vi "AxisControl.vi"() -> ()   [LabVIEW 2020]
uses:
  <vilib>/Utility/miscctls.llb/LVTextColorsTypeDef.ctl
  AxisConfiguration_typedef.ctl
  <vilib>/Modbus/subvis/Modbus API/Modbus API.lvclass/Modbus API.ctl
  <vilib>/Modbus/subvis/Transmission Data Unit (ADU)/Transmission Data Unit/Transmission Data Unit.lvclass/Transmission Data Unit.ctl
  <vilib>/Modbus/master/Data Access/Unit ID/Set Unit ID Property.vi
  <vilib>/Modbus/subvis/Transmission Data Unit (ADU)/Transmission Data Unit/Data Access/Unit ID/Write Unit ID.vi
  <vilib>/Modbus/subvis/Modbus API/Read Transmission Data Unit.vi
  <vilib>/Modbus/subvis/Modbus API/Write Transmission Data Unit.vi
  <vilib>/Modbus/master/Modbus Master.lvclass
  C:/Program Files (x86)/National Instruments/LabVIEW 2020/vi.lib/Modbus/subvis/Modbus API/Modbus API.lvclass
  ConnectionData.vi
  AxisReadValues_Write.vi
  AxisConfiguration.vi
  AxisConfiguration_Write.vi
  AxisWriteValues.vi
  ConnectionData_Write.vi
  AxisReadValues.vi
  <vilib>/Utility/config.llb/Read Key (String).vi
  AxisWriteValues_Write.vi
  <vilib>/Utility/config.llb/Read Key (U32).vi
  <vilib>/Modbus/master/Create Master Instance (Serial).vi
  <vilib>/Modbus/master/Create Master Instance (TCP).vi
  <vilib>/Utility/config.llb/Write Key (String).vi
  <vilib>/Modbus/subvis/Transmission Data Unit (ADU)/Transmission Data Unit/Transmission Data Unit.lvclass
  SMCD14_lib.lvlib
  <vilib>/Utility/config.llb/NI_LVConfig.lvlib
panel:
  out "TimeOut value":u32
  in  "ConnectBtn2":bool
  out "ConnectionStatusIndicator":string="Not connected" caption="Connection status:"
  in  "StopAppBtn":bool caption="Close"
  in  "MainTabs":enum32{"Axis", "Connection", "Config."}(tab)
  out "AxisVelIndicator":sgl caption="Velocity [mm/s]" format="%.4g"
  out "MotorIndicator":bool caption="Motor ON"
  in  "ClearBtn":bool
  in  "StopBtn":bool caption="Stop"
  in  "RunBtn":bool caption="Run"
  in  "VelocityControl":dbl=1.0 caption="Target velocity" min=-50.0 max=50.0 step=1.0
  in  "TargetControl":dbl caption="Target position"
  in  "MoveModeControl":u16(ring)=4 caption="Movement mode" items=["Absolute"=1, "Relative"=2, "Velocity"=3, "Homing"=4, "none"=0]
  out "ErrorCodeIndicator":string="No error" caption="Error description"
  out "AxisPosIndicator":sgl caption="Position [mm]" format="%.4f"
  in  "MotorONBtn":bool
  in  "MotorOFFBtn":bool
  out "IsHomedIndicator":bool caption="Homed"
  out "IsRunningIndicator":bool caption="Running"
  out "FLSIndicator":bool caption="FLS (limit+)"
  out "BLSIndicator":bool caption="BLS (limit-)"
  out "InPosIndicator":bool caption="In position"
  out "EnabledIndicator":bool caption="Enabled"
  out "ErrorIndicator":bool caption="Error"
  out "RefIndicator":bool caption="Ref. signal"
  in  "ReadOnlyMode":bool
  in  "CheckProg":bool
  in  "BaudrateCtrl":u16=38400 caption="Baud rate"
  in  "IPCtrl":string caption="IP address"
  in  "ConnectBtn":bool
  in  "COMportCtrl":refnum<visa-resource-name> caption="COM port"
  in  "ProtocolCtrl":u16(ring) caption="Protocol" items=["Serial", "TCP/IP"]
  in  "DeviceIDCtrl":u16=1 caption="Device ID"
  in  "IsSubPanel":bool
  in  "default config file":string="defaults.ini"
  in  "SubPanelNo":u16=1 caption="SubPanelNo (0-5)"
  in  "Joystick control":bool
  in  "LogIn":bool
  in  "AxisName":string caption="Axis name"
  in  "WriteFileBtn":bool caption="Run"
  in  "ReadFileBtn":bool caption="Run"
  in  "WriteConfBtn":bool caption="Run"
  in  "ReadConfBtn":bool caption="Run"
  in  "UnitsControl":u16(ring) caption="Units" items=["mm", "°"]
  in  "AccDeccControl":dbl=30.0 caption="Acc./dec."
  in  "HomingVelControl":dbl=1.0 caption="Homing velocity"
  in  "OffsetControl":dbl caption="Offset"
  in  "GainControl":dbl=1.0 caption="Gain (gear)"
  in  "BacklashControl":dbl=0.1 caption="Backlash distance"
  in  "HomingTypeControl":u16(ring)=4 caption="Homing type" items=["no homing"=0, "forward limit switch"=1, "backward limit switch"=2, "forward reference"=4, "backward reference"=8]
  in  "JoyMaxSpeed":dbl caption="Joystick max speed"
  in  "JoyMinSpeed":dbl caption="Joystick min. speed"
  in  "Max Velocity":dbl caption="Max. Velocity"
  # "Advanced"
  # "Display settings"
  # "Device settings"
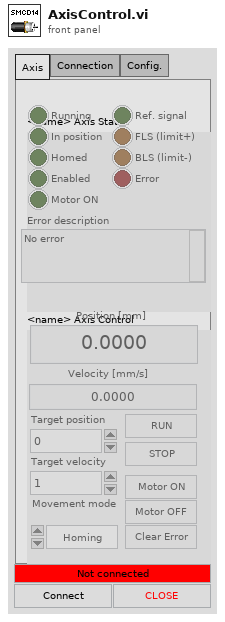
[diagram p1: front panel]
types:
  T1 = typedef "NI_LVConfig.lvlib/Config Data RefNum.ctl" = refnum<k1>
  T2 = typedef "SMCD14_lib.lvlib/AxisConfiguration_typedef.ctl" = cluster{"AxisHomeType":u16, "AxisBacklash":dbl, "AxisGain":dbl, "AxisOffset":dbl, "AxisUnit":u16, "ReqConfRead":bool, "ReqConfWrite":bool, "AxisName":string, "AxisAccDecc":dbl, "AxisHomeVel":dbl}
  T3 = cluster{"Joy_slow_speed":sgl, "Joy_slow_fast":sgl, "Name":string, "UnitsControl":u16, "MaxVel":sgl, "Joystick_control":bool}
  T4 = cluster{"DeviceIDCtrl":u16, "ProtocolCtrl":enum16{"Modbus RTU", "Modbus TCP", ""}, "COMportCtrl":refnum<visa-resource-name>, "IPCtrl":string}
  T5 = typedef "SMCD14_lib.lvlib/AxisWriteValues_typedef.ctl" = cluster{"AxisTarget":dbl, "AxisTargetVel":dbl, "AxisStartReq":bool, "AxisStopReq":bool, "AxisClearReq":bool, "AxisMovetype":bool, "AxisMotorON":bool, "MoveModeControl":u16, "AxisHomingVel":dbl, "AxisAccDecc":dbl}
  T6 = enum8{"Enabled", "Disabled", "Disabled and Grayed Out"}
  T7 = cluster{"Joy_slow_speed":dbl, "Joy_slow_fast":dbl, "Name":string, "UnitsControl":u16, "MaxVel":dbl}
  T8 = typedef "SMCD14_lib.lvlib/ConnectionData_typedef.ctl" = cluster{"DeviceIDCtrl":u16, "ProtocolCtrl":enum16{"Modbus RTU", "Modbus TCP", ""}, "COMportCtrl":refnum<visa-resource-name>, "IPCtrl":string, "serial master instance":refnum<class "Modbus Master.lvclass">, "ConnectionStatusIndicator":bool}
  T9 = typedef "SMCD14_lib.lvlib/AxisReadValues_typedef.ctl" = cluster{"AxisPosition":dbl, "AxisStatus":i16, "AxisErrorCode":i16, "AxisInPos":bool, "AxisRun":bool, "AxisHomed":bool, "AxisFLS":bool, "AxisBLS":bool, "AxisEnabled":bool, "AxisError":bool, "AxisDog":bool, "AxisVelocity":dbl, "AxisHeartbeat":i16, "SICStatus":i16, "AxisMotorON":bool}
  T10 = enum32{"invalid app kind", "Development System", "Run Time System", "Student Edition", "Embedded LabVIEW", "Evaluation", "Custom"}
  T11 = typedef "LVTextColorsTypeDef.ctl" = cluster{"Text Color":u32, "Background Color":u32}
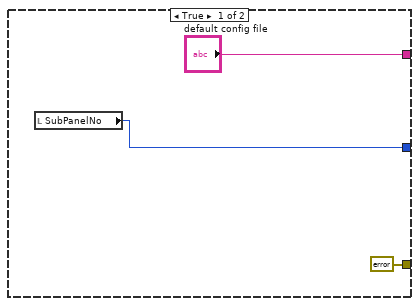
[diagram p2: hidden frame]
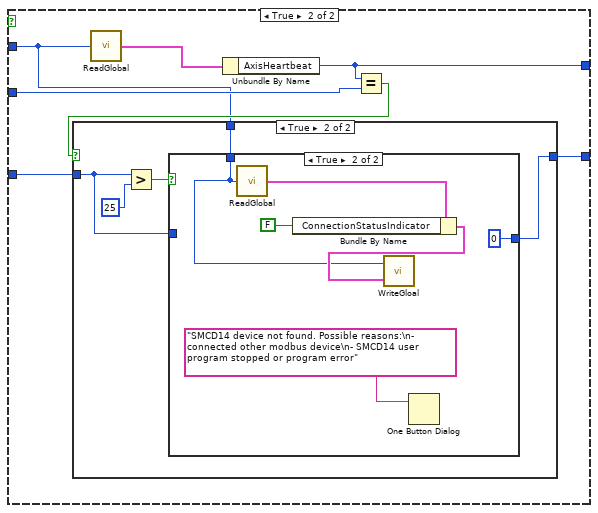
[diagram p3: hidden frame]
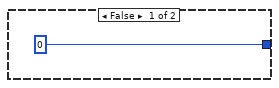
[diagram p4: hidden frame]
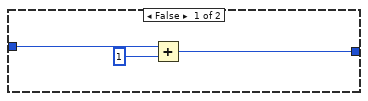
[diagram p5: hidden frame]
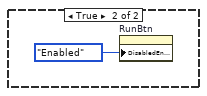
[diagram p6: hidden frame]
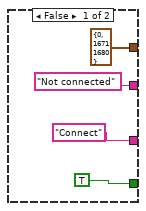
[diagram p7: hidden frame]
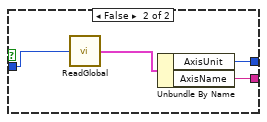
[diagram p8: hidden frame]
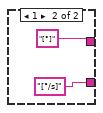
[diagram p9: hidden frame]
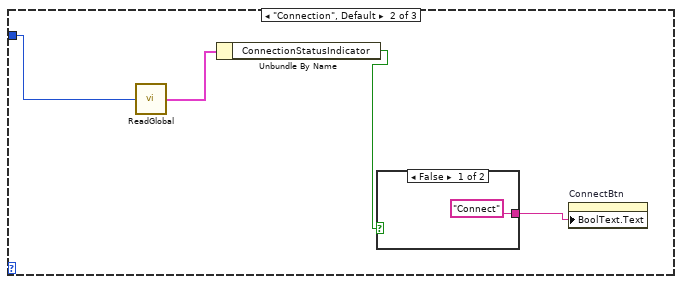
[diagram p10: hidden frame]
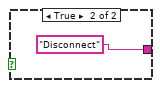
[diagram p11: hidden frame]
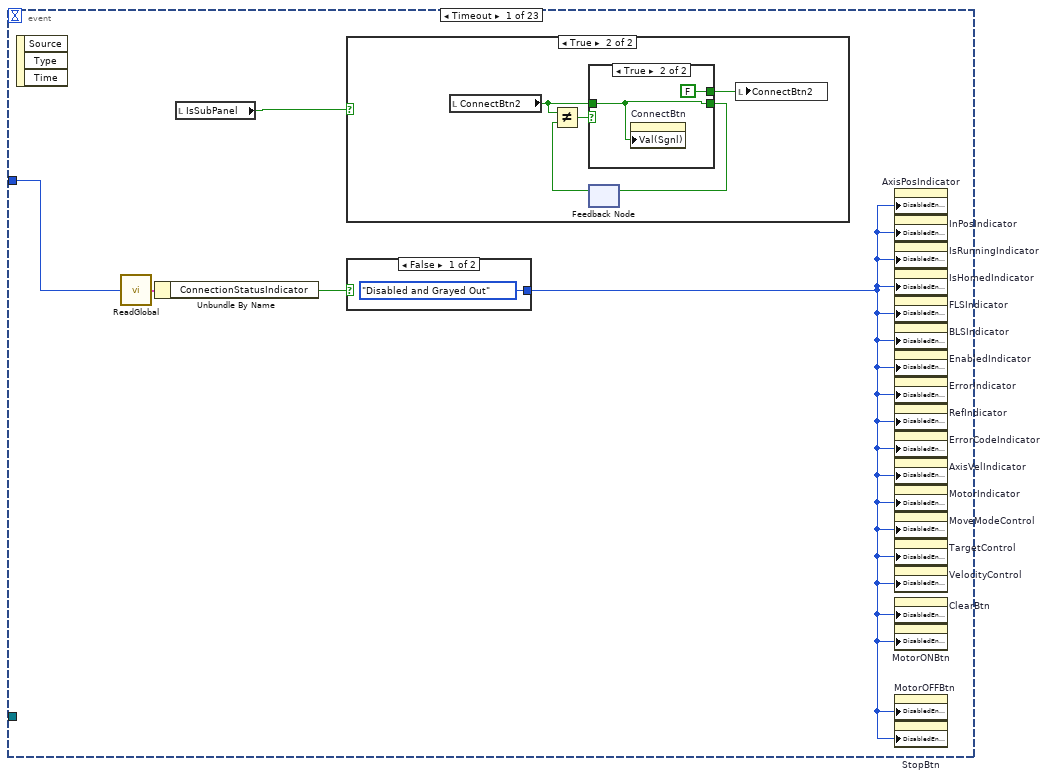
[diagram p13: hidden frame]
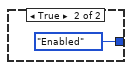
[diagram p14: hidden frame]
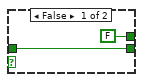
[diagram p16: hidden frame]
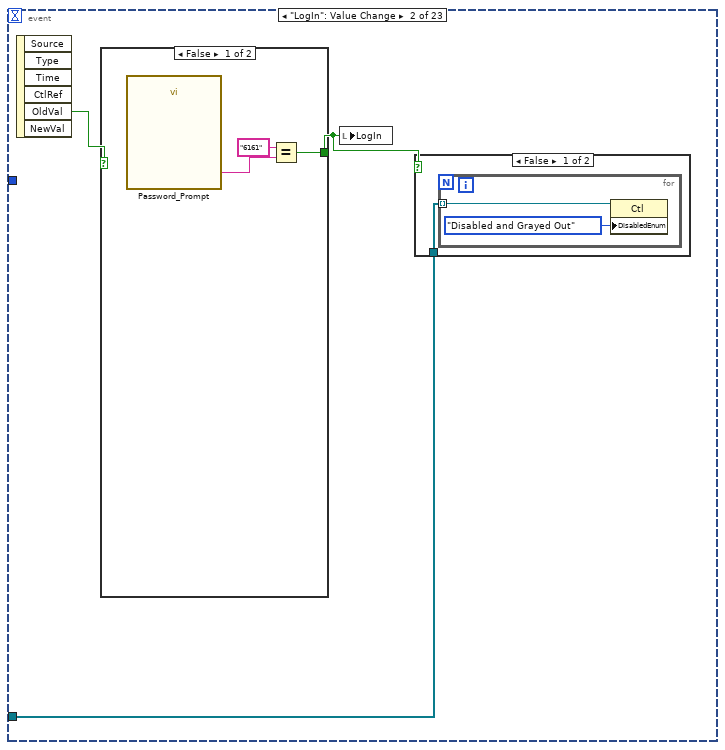
[diagram p17: hidden frame]
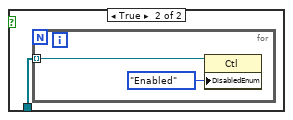
[diagram p18: hidden frame]
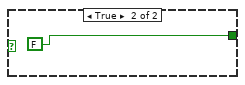
[diagram p19: hidden frame]
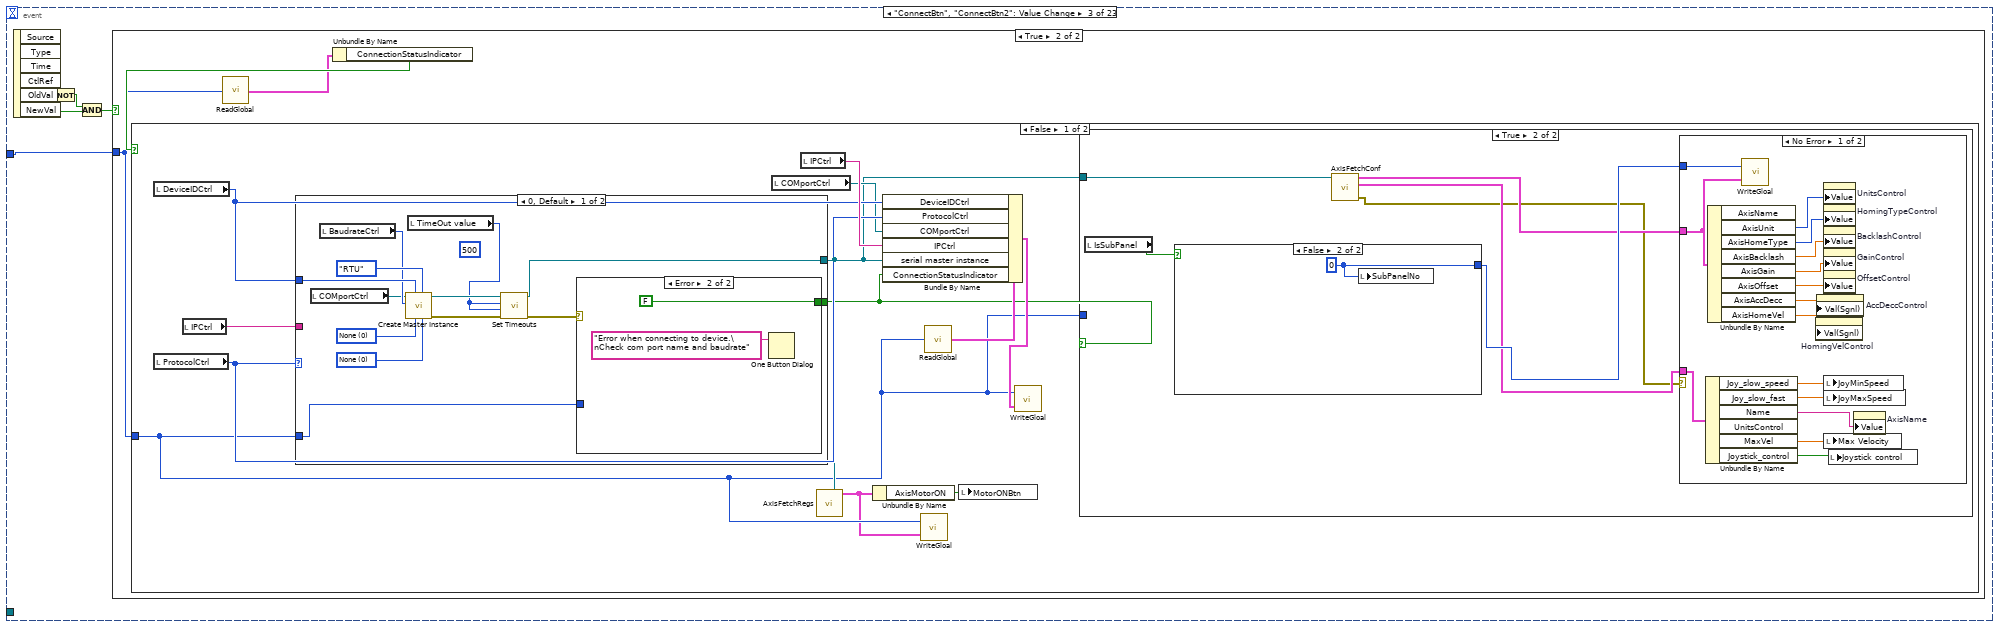
[diagram p20: hidden frame]
diagram:
  # "Wczytanie ustawień domyślnych z pliku defaults.ini w aktualnym folderze"
  # "Wspólne"
  # "Zakładka Configuration"
  # "Zakładka Axis"
  # "Zakładka Connection"
  n1 = local read "IsSubPanel"() -> (w4:bool)
  n2 = case shown="False" w4 {
    tunnel: ["default config file" w41] -> w13
    tunnel: [errorcluster {"status"=FALSE, "code"=0, "source"=""} ("error out") w38] -> w12
    tunnel: [w33 w36] -> w3
    frame True {
      n3 = local read "SubPanelNo"() -> (w33:u16)
    }
    frame False {
      w36 = 0
      n4 = call <vilib>:"Application Directory.vi"() -> ("Application Directory"=w48:path)
      n5 = local write "SubPanelNo"(w36) -> ()
      n6 = Build Path(base path=w48, name or relative path="SMCD14AxisControl.ini") -> (appended path=w46:path)
      n7 = call <vilib>:"Open Config Data.vi"("create file if necessary (T)"=TRUE, "configuration file path"=w46) -> ("error out"=w37:errorcluster, "refnum"=w45:T1)  [unwired: 7 in, 1 out]
      n8 = call-poly <vilib>:"Read Key.vi"("section"="default", "error in (no error)"=w37, "default value"="defaults.ini", "key"="ConfigFile", "refnum"=w45) -> ("error out"=w39:errorcluster, "value"=w41:string, "refnum out"=w40:T1)  [unwired: 3 in, 1 out]
      n9 = call <vilib>:"Close Config Data.vi"("error in (no error)"=w39, "refnum"=w40) -> ("error out"=w38:errorcluster)  [unwired: 8 in, 1 out]
    }
  }
  n10 = Not(x=w4) -> (.not. x?=w2:bool)
  n11 = property on="StopAppBtn" class="Bool (strict)"("Visible"=w2) -> ()  [unwired: 2 in, 2 out]
  n12 = property on="ConnectBtn2" class="Bool (strict)"("Visible"=w2) -> ()  [unwired: 2 in, 2 out]
  n13 = flat-sequence {
    tunnel: w13 -> [w76]
    tunnel: w12 -> [w75]
    tunnel: [w74] -> w11
    tunnel: [w60] -> w5
    tunnel: w3 -> [w52]
    frame #0 {
      n14 = call <vilib>:"Application Directory.vi"() -> ("Application Directory"=w79:path)
      n15 = call <vilib>:"Clear Errors.vi"("error in (no error)"=w75) -> ()  [unwired: 5 in, 2 out]
      n16 = Build Path(base path=w79, name or relative path=w76) -> (appended path=w74:path)
      n17 = call-poly "ReadGlobal.vi"("AxisNo"=w52) -> ("AxisConfigurationOUT"=w57:T2)
      n18 = call "AxisGetConfFromFile.vi"("conf file path"=w74, "AxisConfigurationIn"=w57) -> ("error out"=w60:errorcluster, "AditionalConfigOut"=w73:T3, "AxisConfigurationOut"=w56:T2, "Comunication"=w51:T4)  [unwired: 5 in, 1 out]
      n19 = call-poly "WriteGloal.vi"("AxisConfigurationIN"=w56, "AxisNo"=w52) -> ()  [unwired: 1 in]
      n20 = Unbundle By Name(w73) -> ("Joy_slow_speed"=w59:sgl, "Joy_slow_fast"=w58:sgl, "MaxVel"=w66:sgl, "Joystick_control"=w50:bool)  [unwired: 2 out]
      n21 = Unbundle By Name(w51) -> ("DeviceIDCtrl"=w72:u16, "ProtocolCtrl"=w71:enum16{"Modbus RTU", "Modbus TCP", ""}, "COMportCtrl"=w70:refnum<visa-resource-name>, "IPCtrl"=w69:string)
      n22 = Unbundle By Name(w56) -> ("AxisHomeType"=w65:u16, "AxisBacklash"=w64:dbl, "AxisGain"=w63:dbl, "AxisOffset"=w62:dbl, "AxisUnit"=w67:u16, "AxisName"=w68:string, "AxisAccDecc"=w61:dbl, "AxisHomeVel"=w53:dbl)  [unwired: 2 out]
      n23 = property on="DeviceIDCtrl" class="DigNum (strict)"("Value"=w72) -> ()  [unwired: 2 in, 2 out]
      n24 = property on="ProtocolCtrl" class="Ring (strict)"("Value"=w71) -> ()  [unwired: 2 in, 2 out]
      n25 = property on="COMportCtrl" class="VISAName"("Value"=w70) -> ()  [unwired: 2 in, 2 out]
      n26 = property on="IPCtrl" class="Str"("Value"=w69) -> ()  [unwired: 2 in, 2 out]
      n27 = property on="HomingTypeControl" class="Ring (strict)"("Value"=w65) -> ()  [unwired: 2 in, 2 out]
      n28 = property on="GainControl" class="DigNum (strict)"("Value"=w63) -> ()  [unwired: 2 in, 2 out]
      n29 = property on="UnitsControl" class="Ring (strict)"("Value"=w67) -> ()  [unwired: 2 in, 2 out]
      n30 = property on="AxisName" class="Str"("Value"=w68) -> ()  [unwired: 2 in, 2 out]
      n31 = property on="HomingVelControl" class="DigNum (strict)"("Value"=w53) -> ()  [unwired: 2 in, 2 out]
      n32 = local write "Joystick control"(w50) -> ()
      n33 = local write "JoyMinSpeed"(w59) -> ()
      n34 = local write "JoyMaxSpeed"(w58) -> ()
      n35 = call-poly "ReadGlobal.vi"("AxisNo"=w52) -> ("AxisWriteValuesOUT"=w54:T5)
      n36 = Bundle By Name(cluster=w54, "AxisAccDecc"=w53) -> (w55:T5)
      n37 = Absolute Value(x=w66) -> (abs(x)=w77:sgl)
      n38 = Negate(x=w77) -> (-x=w78:sgl)
      n39 = local write "Max Velocity"(w77) -> ()
      n40 = property on="BacklashControl" class="DigNum (strict)"("Value"=w64) -> ()  [unwired: 2 in, 2 out]
      n41 = property on="OffsetControl" class="DigNum (strict)"("Value"=w62) -> ()  [unwired: 2 in, 2 out]
      n42 = property on="AccDeccControl" class="DigNum (strict)"("Value"=w61) -> ()  [unwired: 2 in, 2 out]
      n43 = property on="VelocityControl" class="DigNum (strict)"("Maximum"=w77, "Minimum"=w78) -> ()  [unwired: 2 in, 2 out]
      n44 = call-poly "WriteGloal.vi"("AxisWriteValuesIN"=w55, "AxisNo"=w52) -> ()  [unwired: 1 in]
    }
  }
  n45 = control-ref of="Joystick control"() -> (w1:refnum<vi>)
  n46 = control-ref of="JoyMinSpeed"() -> (w19:refnum<vi>)
  n47 = control-ref of="JoyMaxSpeed"() -> (w20:refnum<vi>)
  n48 = control-ref of="AccDeccControl"() -> (w21:refnum<vi>)
  n49 = control-ref of="HomingVelControl"() -> (w22:refnum<vi>)
  n50 = control-ref of="OffsetControl"() -> (w23:refnum<vi>)
  n51 = control-ref of="GainControl"() -> (w24:refnum<vi>)
  n52 = control-ref of="BacklashControl"() -> (w25:refnum<vi>)
  n53 = control-ref of="WriteConfBtn"() -> (w26:refnum<vi>)
  n54 = control-ref of="HomingTypeControl"() -> (w17:refnum<vi>)
  n55 = control-ref of="UnitsControl"() -> (w16:refnum<vi>)
  n56 = control-ref of="Max Velocity"() -> (w15:refnum<vi>)
  n57 = control-ref of="AxisName"() -> (w14:refnum<vi>)
  n58 = call <vilib>:"Open Config Data.vi"("error in (no error)"=w5, "create file if necessary (T)"=TRUE, "configuration file path"=w11) -> ("error out"=w9:errorcluster, "refnum"=w10:T1)  [unwired: 6 in, 1 out]
  n59 = Build Array(w19, w20, w21, w22, w23, w24, w25, w26, w17, w16, w15, w14, w1) -> (w18:refnum<vi>[])
  n60 = local write "LogIn"(FALSE ("LogIn")) -> ()
  n61 = call-poly <vilib>:"Read Key.vi"("section"="default", "error in (no error)"=w9, "default value"=u32 1000, "key"="TimeOut", "refnum"=w10) -> ("error out"=w8:errorcluster, "value"=→"TimeOut value":u32, "refnum out"=w7:T1)  [unwired: 3 in, 1 out]
  n62 = for {
    tunnel: w18 -> [w81] mode=indexing
    n63 = property class="Ctl"(reference=w81, "DisabledEnum"=T6."Disabled and Grayed Out" ("Disabled")) -> ()  [unwired: 1 in, 2 out]
  }
  n64 = call <vilib>:"Close Config Data.vi"("error in (no error)"=w8, "refnum"=w7) -> ("error out"=w6:errorcluster)  [unwired: 8 in, 1 out]
  n65 = call <vilib>:"Clear Errors.vi"("error in (no error)"=w6) -> ()  [unwired: 5 in, 2 out]
  n66 = while "ButtonsActions" {
    tunnel: w18 -> [w83]
    stop <- w84 stop-if-true
    n67 = local read "SubPanelNo"() -> (w82:u16)
    n68 = event shown="[8] \"WriteConfBtn\": Value Change" {
      selector: _ -> [_ _ _ _ _ _ _ _ _ _ _ _ _ _ _ _ _ _ _ _ _ _ _]
      dyn-events: _ -> [_ _ _ _ _ _ _ _ _ _ _ _ _ _ _ _ _ _ _ _ _ _ _]
      timeout: 5 -> [_ _ _ _ _ _ _ _ _ _ _ _ _ _ _ _ _ _ _ _ _ _ _]
      tunnel: w83 -> [_ w103 _ _ _ _ _ _ _ _ _ _ _ _ _ _ _ _ _ _ _ _ _]
      tunnel: w82 -> [w89 _ w115 w199 w204 w210 w228 w246 w255 w270 _ w296 w329 w383 w429 w439 w443 w447 w451 w455 w459 w463 w467]
      event Timeout {
        n69 = event-data() -> ()  [unwired: 1 in, 3 out]
        n70 = call-poly "ReadGlobal.vi"("AxisNo"=w89) -> ("ConnectionDataOUT"=w88:T8)
        n71 = Unbundle By Name(w88) -> ("ConnectionStatusIndicator"=w87:bool)
        n72 = local read "IsSubPanel"() -> (w90:bool)
        n73 = case shown="True" w90 {
          frame False {
          }
          frame True {
            n74 = local read "ConnectBtn2"() -> (w94:bool)
            n75 = feedback #1() -> (w97:bool)  [unwired: 1 in]
            n76 = Not Equal?(x=w94, y=w97) -> (x != y?=w95:bool)
            n77 = case shown="True" w95 {
              tunnel: [w99 w101] -> w96
              tunnel: w94 -> [w99 w101]
              tunnel: [FALSE FALSE] -> w93
              frame False {
              }
              frame True {
                n78 = property on="ConnectBtn" class="Bool (strict)"("Val(Sgnl)"=w101) -> ()  [unwired: 2 in, 2 out]
              }
            }
            n79 = feedback-in #1(w96) -> ()
            n80 = local write "ConnectBtn2"(w93) -> ()
          }
        }
        n81 = case shown="False" w87 {
          tunnel: [T6."Disabled and Grayed Out" ("Disabled") T6."Enabled" ("Disabled")] -> w86
          frame False {
          }
          frame True {
          }
        }
        n82 = property on="AxisPosIndicator" class="DigNum (strict)"("DisabledEnum"=w86) -> ()  [unwired: 2 in, 2 out]
        n83 = property on="InPosIndicator" class="Bool (strict)"("DisabledEnum"=w86) -> ()  [unwired: 2 in, 2 out]
        n84 = property on="IsRunningIndicator" class="Bool (strict)"("DisabledEnum"=w86) -> ()  [unwired: 2 in, 2 out]
        n85 = property on="IsHomedIndicator" class="Bool (strict)"("DisabledEnum"=w86) -> ()  [unwired: 2 in, 2 out]
        n86 = property on="FLSIndicator" class="Bool (strict)"("DisabledEnum"=w86) -> ()  [unwired: 2 in, 2 out]
        n87 = property on="BLSIndicator" class="Bool (strict)"("DisabledEnum"=w86) -> ()  [unwired: 2 in, 2 out]
        n88 = property on="EnabledIndicator" class="Bool (strict)"("DisabledEnum"=w86) -> ()  [unwired: 2 in, 2 out]
        n89 = property on="ErrorIndicator" class="Bool (strict)"("DisabledEnum"=w86) -> ()  [unwired: 2 in, 2 out]
        n90 = property on="RefIndicator" class="Bool (strict)"("DisabledEnum"=w86) -> ()  [unwired: 2 in, 2 out]
        n91 = property on="ErrorCodeIndicator" class="Str"("DisabledEnum"=w86) -> ()  [unwired: 2 in, 2 out]
        n92 = property on="AxisVelIndicator" class="DigNum (strict)"("DisabledEnum"=w86) -> ()  [unwired: 2 in, 2 out]
        n93 = property on="MotorIndicator" class="Bool (strict)"("DisabledEnum"=w86) -> ()  [unwired: 2 in, 2 out]
        n94 = property on="MoveModeControl" class="Ring (strict)"("DisabledEnum"=w86) -> ()  [unwired: 2 in, 2 out]
        n95 = property on="TargetControl" class="DigNum (strict)"("DisabledEnum"=w86) -> ()  [unwired: 2 in, 2 out]
        n96 = property on="VelocityControl" class="DigNum (strict)"("DisabledEnum"=w86) -> ()  [unwired: 2 in, 2 out]
        n97 = property on="ClearBtn" class="Bool (strict)"("DisabledEnum"=w86) -> ()  [unwired: 2 in, 2 out]
        n98 = property on="MotorONBtn" class="Bool (strict)"("DisabledEnum"=w86) -> ()  [unwired: 2 in, 2 out]
        n99 = property on="MotorOFFBtn" class="Bool (strict)"("DisabledEnum"=w86) -> ()  [unwired: 2 in, 2 out]
        n100 = property on="StopBtn" class="Bool (strict)"("DisabledEnum"=w86) -> ()  [unwired: 2 in, 2 out]
      }
      event "LogIn": Value Change {
        n101 = event-data() -> ("OldVal"=w104:bool)  [unwired: 1 in, 5 out]
        n102 = case shown="False" w104 {
          tunnel: [w111 FALSE ("LogIn")] -> w102
          frame False {
            n103 = call "Password_Prompt.vi"() -> ("Password"=w113:string)  [unwired: 17 in, 2 out]
            n104 = Equal?(x="6161", y=w113) -> (x = y?=w111:bool)
          }
          frame True {
          }
        }
        n105 = local write "LogIn"(w102) -> ()
        n106 = case shown="False" w102 {
          tunnel: w103 -> [w105 w108]
          frame False {
            n107 = for {
              tunnel: w105 -> [w107] mode=indexing
              n108 = property class="Ctl"(reference=w107, "DisabledEnum"=T6."Disabled and Grayed Out" ("Disabled")) -> ()  [unwired: 1 in, 2 out]
            }
          }
          frame True {
            n109 = for {
              tunnel: w108 -> [w110] mode=indexing
              n110 = property class="Ctl"(reference=w110, "DisabledEnum"=T6."Enabled" ("Disabled")) -> ()  [unwired: 1 in, 2 out]
            }
          }
        }
      }
      event "ConnectBtn", "ConnectBtn2": Value Change {
        n111 = event-data() -> ("OldVal"=w117:bool, "NewVal"=w118:bool)  [unwired: 1 in, 4 out]
        n112 = Not(x=w117) -> (.not. x?=w116:bool)
        n113 = And(x=w116, y=w118) -> (x .and. y?=w119:bool)
        n114 = case shown="True" w119 {
          tunnel: w115 -> [_ w120]
          frame False {
          }
          frame True {
            n115 = call-poly "ReadGlobal.vi"("AxisNo"=w120) -> ("ConnectionDataOUT"=w121:T8)
            n116 = Unbundle By Name(w121) -> ("ConnectionStatusIndicator"=w122:bool)
            n117 = case shown="False" w122 {
              tunnel: w120 -> [w124 w193]
              frame False {
                n118 = local read "DeviceIDCtrl"() -> (w132:u16)
                n119 = local read "ProtocolCtrl"() -> (w133:u16)
                n120 = local read "IPCtrl"() -> (w131:string)
                n121 = case shown="0, Default" w133 {
                  tunnel: w132 -> [w170 w179]
                  tunnel: [w163 w180] -> w125
                  tunnel: [w164 w184] -> w127
                  tunnel: w131 -> [_ w188]
                  tunnel: w124 -> [w158 _]
                  frame 0, Default {
                    (unwired) 500 ("read operation timeout (ms)")
                    w165 = u16 0 items=["None", "XON/XOFF", "RTS/CTS", "XON/XOFF & RTS/CTS", "DTR/DSR", "XON/XOFF & DTR/DSR"] ("flow control (None)")
                    w166 = u16 0 items=["None", "Odd", "Even"] ("parity (Even)")
                    n122 = local read "COMportCtrl"() -> (w159:refnum<visa-resource-name>)
                    n123 = local read "BaudrateCtrl"() -> (w161:u16)
                    n124 = call-poly <vilib>:"Create Master Instance.vi"("flow control (None)"=w165, "serial type"=enum16{"RTU", "ASCII"}."RTU", "parity (Even)"=w166, "unit ID"=w170, "baud rate (9600)"=w161, "VISA resource name"=w159) -> ("error out"=w167:errorcluster, "serial master instance"=w168:refnum<class "Modbus Master.lvclass">)  [unwired: 4 in]
                    n125 = local read "TimeOut value"() -> (w160:u32)
                    n126 = call <vilib>:"Set Timeouts.vi"("error in (no error)"=w167, "write operation timeout (ms)"=w160, "read operation timeout (ms)"=w160, "Modbus master in"=w168) -> ("error out"=w162:errorcluster, "Modbus master out"=w163:refnum<class "Modbus Master.lvclass">)  [unwired: 6 in]
                    n127 = case shown="Error" w162 {
                      tunnel: [TRUE ("ConnectionStatusIndicator") FALSE ("ConnectionStatusIndicator")] -> w164
                      tunnel: w158 -> [w172 _]
                      frame No Error {
                        n128 = Bundle By Name(cluster=T2 {"AxisHomeType"=4, "AxisBacklash"=0.699999988079071, "AxisGain"=6.0, "AxisOffset"=0.0, "AxisUnit"=0, "ReqConfRead"=FALSE, "ReqConfWrite"=FALSE, "AxisName"="", "AxisAccDecc"=0.0, "AxisHomeVel"=0.0} ("AxisConfiguration"), "ReqConfRead"=TRUE) -> (w171:T2)
                        n129 = call-poly "WriteGloal.vi"("AxisConfigurationIN"=w171, "AxisNo"=w172) -> ()  [unwired: 1 in]
                      }
                      frame Error {
                        n130 = One Button Dialog(message="Error when connecting to device.\nCheck com port name and baudrate") -> ()  [unwired: 1 in, 1 out]
                      }
                    }
                  }
                  frame 1 {
                    (unwired) 500 ("read operation timeout (ms)")
                    n131 = local read "TimeOut value"() -> (w178:u32)
                    n132 = call-poly <vilib>:"Create Master Instance.vi"("port (502)"=u16 502, "address"=w188) -> ("error out"=w185:errorcluster, "TCP master instance"=w186:refnum<class "Modbus Master.lvclass">)  [unwired: 8 in]
                    n133 = call <vilib>:"Set Timeouts.vi"("error in (no error)"=w185, "write operation timeout (ms)"=w178, "read operation timeout (ms)"=w178, "Modbus master in"=w186) -> ("error out"=w182:errorcluster, "Modbus master out"=w183:refnum<class "Modbus Master.lvclass">)  [unwired: 6 in]
                    n134 = call <vilib>:"Set Unit ID.vi"("error in (no error)"=w182, "unit ID"=w179, "Modbus master in"=w183) -> ("error out"=w181:errorcluster, "Modbus master out"=w180:refnum<class "Modbus Master.lvclass">)  [unwired: 7 in]
                    n135 = case shown="No Error" w181 {
                      tunnel: [TRUE ("ConnectionStatusIndicator") FALSE ("ConnectionStatusIndicator")] -> w184
                      frame No Error {
                      }
                      frame Error {
                        n136 = One Button Dialog(message="Error when connecting to device.\nCheck ip adress or network settings.") -> ()  [unwired: 1 in, 1 out]
                      }
                    }
                  }
                }
                n137 = local read "COMportCtrl"() -> (w130:refnum<visa-resource-name>)
                n138 = local read "IPCtrl"() -> (w134:string)
                n139 = call "AxisFetchRegs.vi"("Modbus master"=w125) -> ("AxisReadValues"=w123:T9)  [unwired: 8 in, 2 out]
                n140 = Unbundle By Name(w123) -> ("AxisMotorON"=w126:bool)
                n141 = call-poly "WriteGloal.vi"("AxisReadValuesIN"=w123, "AxisNo"=w124) -> ()  [unwired: 1 in]
                n142 = call-poly "ReadGlobal.vi"("AxisNo"=w124) -> ("ConnectionDataOUT"=w128:T8)
                n143 = Bundle By Name(cluster=w128, "DeviceIDCtrl"=w132, "ProtocolCtrl"=w133, "COMportCtrl"=w130, "IPCtrl"=w134, "serial master instance"=w125, "ConnectionStatusIndicator"=w127) -> (w129:T8)
                n144 = local write "MotorONBtn"(w126) -> ()
                n145 = call-poly "WriteGloal.vi"("ConnectionDataIN"=w129, "AxisNo"=w124) -> ()  [unwired: 1 in]
                n146 = case shown="True" w127 {
                  tunnel: w124 -> [_ _]
                  tunnel: w125 -> [_ w138]
                  frame False {
                  }
                  frame True {
                    n147 = local read "IsSubPanel"() -> (w139:bool)
                    n148 = case shown="False" w139 {
                      tunnel: [w156 w157] -> w140
                      frame True {
                        n149 = local read "SubPanelNo"() -> (w156:u16)
                      }
                      frame False {
                        w157 = 0
                        n150 = local write "SubPanelNo"(w157) -> ()
                      }
                    }
                    n151 = call "AxisFetchConf.vi"("Modbus master"=w138) -> ("error out"=w135:errorcluster, "JoyControl"=w137:T3, "AxisConfiguration"=w136:T2)  [unwired: 8 in]
                    n152 = case shown="No Error" w135 {
                      tunnel: w136 -> [w146 _]
                      tunnel: w137 -> [w150 _]
                      tunnel: w140 -> [w145 _]
                      frame No Error {
                        n153 = Unbundle By Name(w150) -> ("Joy_slow_speed"=w147:sgl, "Joy_slow_fast"=w148:sgl, "Name"=w141:string, "MaxVel"=w149:sgl, "Joystick_control"=w144:bool)  [unwired: 1 out]
                        n154 = Unbundle By Name(w146) -> ("AxisUnit"=w155:u16, "AxisHomeType"=w154:u16, "AxisBacklash"=w153:dbl, "AxisGain"=w152:dbl, "AxisOffset"=w151:dbl, "AxisAccDecc"=w143:dbl, "AxisHomeVel"=w142:dbl)  [unwired: 1 out]
                        n155 = call-poly "WriteGloal.vi"("AxisConfigurationIN"=w146, "AxisNo"=w145) -> ()  [unwired: 1 in]
                        n156 = property on="HomingVelControl" class="DigNum (strict)"("Val(Sgnl)"=w142) -> ()  [unwired: 2 in, 2 out]
                        n157 = property on="AccDeccControl" class="DigNum (strict)"("Val(Sgnl)"=w143) -> ()  [unwired: 2 in, 2 out]
                        n158 = property on="UnitsControl" class="Ring (strict)"("Value"=w155) -> ()  [unwired: 2 in, 2 out]
                        n159 = property on="HomingTypeControl" class="Ring (strict)"("Value"=w154) -> ()  [unwired: 2 in, 2 out]
                        n160 = property on="BacklashControl" class="DigNum (strict)"("Value"=w153) -> ()  [unwired: 2 in, 2 out]
                        n161 = property on="GainControl" class="DigNum (strict)"("Value"=w152) -> ()  [unwired: 2 in, 2 out]
                        n162 = property on="OffsetControl" class="DigNum (strict)"("Value"=w151) -> ()  [unwired: 2 in, 2 out]
                        n163 = local write "JoyMinSpeed"(w147) -> ()
                        n164 = local write "JoyMaxSpeed"(w148) -> ()
                        n165 = local write "Max Velocity"(w149) -> ()
                        n166 = local write "Joystick control"(w144) -> ()
                        n167 = property on="AxisName" class="Str"("Value"=w141) -> ()  [unwired: 2 in, 2 out]
                      }
                      frame Error {
                      }
                    }
                  }
                }
              }
              frame True {
                n168 = call-poly "ReadGlobal.vi"("AxisNo"=w193) -> ("ConnectionDataOUT"=w194:T8)
                n169 = Bundle By Name(cluster=w194, "ConnectionStatusIndicator"=FALSE) -> (w192:T8)
                n170 = call-poly "WriteGloal.vi"("ConnectionDataIN"=w192, "AxisNo"=w193) -> ()  [unwired: 1 in]
                n171 = Unbundle By Name(w192) -> ("serial master instance"=w195:refnum<class "Modbus Master.lvclass">)
                n172 = call-dynamic "Close.vi"("Modbus master in"=w195) -> ()  [unwired: 10 in, 1 out]
              }
            }
          }
        }
      }
      event Panel Close? {
        n173 = event-data() -> ()  [unwired: 1 in, 4 out]
        n174 = disable-structure shown="Disabled" {
          disable-tunnel: w199 -> [w202 _]
          frame Disabled {
            n175 = call-poly "ReadGlobal.vi"("AxisNo"=w202) -> ("ConnectionDataOUT"=w201:T8)
            n176 = Unbundle By Name(w201) -> ("serial master instance"=w203:refnum<class "Modbus Master.lvclass">)
            n177 = call-dynamic "Close.vi"("Modbus master in"=w203) -> ()  [unwired: 10 in, 1 out]
          }
          frame Enabled {
          }
        }
        n178 = call-poly "ReadGlobal.vi"("AxisNo"=w199) -> ("ConnectionDataOUT"=w200:T8)
        n179 = Bundle By Name(cluster=w200, "ConnectionStatusIndicator"=FALSE) -> (w198:T8)
        n180 = call-poly "WriteGloal.vi"("ConnectionDataIN"=w198, "AxisNo"=w199) -> ()  [unwired: 1 in]
        n181 = event-data() -> ()  [unwired: 2 in, 1 out]
      }
      event "StopAppBtn": Value Change {
        n182 = event-data() -> ()  [unwired: 1 in, 6 out]
        n183 = call-poly "ReadGlobal.vi"("AxisNo"=w204) -> ("ConnectionDataOUT"=w207:T8)
        n184 = Open VI Reference(vi path=path "AxisControl.vi") -> (vi reference=w208:refnum<vi>)  [unwired: 5 in, 1 out]
        n185 = Bundle By Name(cluster=w207, "ConnectionStatusIndicator"=FALSE) -> (w206:T8)
        n186 = call-poly "WriteGloal.vi"("ConnectionDataIN"=w206, "AxisNo"=w204) -> ()  [unwired: 1 in]
        n187 = invoke class="VI" method="Abort VI"(reference=w208) -> ()  [unwired: 2 in, 3 out]
      }
      event "ClearBtn": Value Change {
        n188 = event-data() -> ("OldVal"=w214:bool, "NewVal"=w212:bool)  [unwired: 1 in, 4 out]
        n189 = Not(x=w214) -> (.not. x?=w213:bool)
        n190 = And(x=w213, y=w212) -> (x .and. y?=w211:bool)
        n191 = case shown="True" w211 {
          tunnel: w210 -> [_ w217]
          frame False {
          }
          frame True {
            n192 = flat-sequence {
              tunnel: w217 -> [w218]
              tunnel: [w218] -> w215
              tunnel: [w222] -> w216
              tunnel: w215 -> [w222]
              tunnel: w216 -> [w224]
              frame #0 {
                n193 = call-poly "ReadGlobal.vi"("AxisNo"=w218) -> ("AxisWriteValuesOUT"=w220:T5)
                n194 = Bundle By Name(cluster=w220, "AxisClearReq"=TRUE ("AxisWriteValues.AxisMotorON")) -> (w219:T5)
                n195 = call-poly "WriteGloal.vi"("AxisWriteValuesIN"=w219, "AxisNo"=w218) -> ()  [unwired: 1 in]
              }
              frame #1 {
                n196 = Wait (ms)(milliseconds to wait=u32 500) -> ()  [unwired: 1 out]
              }
              frame #2 {
                n197 = call-poly "ReadGlobal.vi"("AxisNo"=w224) -> ("AxisWriteValuesOUT"=w226:T5)
                n198 = Bundle By Name(cluster=w226, "AxisClearReq"=FALSE ("AxisWriteValues.AxisMotorON")) -> (w225:T5)
                n199 = call-poly "WriteGloal.vi"("AxisWriteValuesIN"=w225, "AxisNo"=w224) -> ()  [unwired: 1 in]
              }
            }
          }
        }
      }
      event "RunBtn": Value Change {
        n200 = event-data() -> ("OldVal"=w232:bool, "NewVal"=w230:bool)  [unwired: 1 in, 4 out]
        n201 = Not(x=w232) -> (.not. x?=w231:bool)
        n202 = And(x=w231, y=w230) -> (x .and. y?=w229:bool)
        n203 = case shown="True" w229 {
          tunnel: w228 -> [_ w235]
          frame False {
          }
          frame True {
            n204 = flat-sequence {
              tunnel: w235 -> [w236]
              tunnel: [w236] -> w234
              tunnel: w234 -> [w240]
              tunnel: [w240] -> w233
              tunnel: w233 -> [w242]
              frame #0 {
                n205 = call-poly "ReadGlobal.vi"("AxisNo"=w236) -> ("AxisWriteValuesOUT"=w238:T5)
                n206 = Bundle By Name(cluster=w238, "AxisStartReq"=TRUE ("AxisWriteValues.AxisMotorON")) -> (w237:T5)
                n207 = call-poly "WriteGloal.vi"("AxisWriteValuesIN"=w237, "AxisNo"=w236) -> ()  [unwired: 1 in]
              }
              frame #1 {
                n208 = Wait (ms)(milliseconds to wait=u32 500) -> ()  [unwired: 1 out]
              }
              frame #2 {
                n209 = call-poly "ReadGlobal.vi"("AxisNo"=w242) -> ("AxisWriteValuesOUT"=w244:T5)
                n210 = Bundle By Name(cluster=w244, "AxisStartReq"=FALSE ("AxisWriteValues.AxisMotorON")) -> (w243:T5)
                n211 = call-poly "WriteGloal.vi"("AxisWriteValuesIN"=w243, "AxisNo"=w242) -> ()  [unwired: 1 in]
              }
            }
          }
        }
      }
      event "ReadConfBtn": Value Change {
        n212 = event-data() -> ("OldVal"=w250:bool, "NewVal"=w248:bool)  [unwired: 1 in, 4 out]
        n213 = Not(x=w250) -> (.not. x?=w249:bool)
        n214 = And(x=w249, y=w248) -> (x .and. y?=w247:bool)
        n215 = case shown="True" w247 {
          tunnel: w246 -> [_ w251]
          frame False {
          }
          frame True {
            n216 = Bundle By Name(cluster=T2 {"AxisHomeType"=4, "AxisBacklash"=0.699999988079071, "AxisGain"=6.0, "AxisOffset"=0.0, "AxisUnit"=0, "ReqConfRead"=FALSE, "ReqConfWrite"=FALSE, "AxisName"="", "AxisAccDecc"=0.0, "AxisHomeVel"=0.0} ("AxisConfiguration"), "ReqConfRead"=TRUE) -> (w252:T2)
            n217 = call-poly "WriteGloal.vi"("AxisConfigurationIN"=w252, "AxisNo"=w251) -> ()  [unwired: 1 in]
          }
        }
      }
      event "WriteConfBtn": Value Change {
        n218 = event-data() -> ("OldVal"=w260:bool, "NewVal"=w258:bool)  [unwired: 1 in, 4 out]
        n219 = Not(x=w260) -> (.not. x?=w259:bool)
        n220 = And(x=w259, y=w258) -> (x .and. y?=w257:bool)
        n221 = case shown="True" w257 {
          selector: w257 -> [w261 w263]
          tunnel: [w261 w262] -> w256
          frame False {
          }
          frame True {
            n222 = Two Button Dialog(message="Do you want to save configuration to driver?") -> (T button?=w264:bool)  [unwired: 2 in]
            n223 = And(x=w264, y=w263) -> (x .and. y?=w262:bool)
          }
        }
        n224 = case shown="True" w256 {
          tunnel: w255 -> [_ w266]
          frame False {
          }
          frame True {
            n225 = Bundle By Name(cluster=T2 {"AxisHomeType"=4, "AxisBacklash"=0.699999988079071, "AxisGain"=6.0, "AxisOffset"=0.0, "AxisUnit"=0, "ReqConfRead"=FALSE, "ReqConfWrite"=FALSE, "AxisName"="", "AxisAccDecc"=0.0, "AxisHomeVel"=0.0} ("AxisConfiguration"), "ReqConfWrite"=TRUE ("ReqConfRead")) -> (w267:T2)
            n226 = call-poly "WriteGloal.vi"("AxisConfigurationIN"=w267, "AxisNo"=w266) -> ()  [unwired: 1 in]
          }
        }
      }
      event "StopBtn": Value Change {
        n227 = event-data() -> ("OldVal"=w274:bool, "NewVal"=w272:bool)  [unwired: 1 in, 4 out]
        n228 = Not(x=w274) -> (.not. x?=w273:bool)
        n229 = And(x=w273, y=w272) -> (x .and. y?=w271:bool)
        n230 = case shown="True" w271 {
          tunnel: w270 -> [_ w277]
          frame False {
          }
          frame True {
            n231 = flat-sequence {
              tunnel: w277 -> [w279]
              tunnel: [w279] -> w276
              tunnel: w276 -> [w282]
              tunnel: [w282] -> w275
              tunnel: w275 -> [w284]
              frame #0 {
                n232 = call-poly "ReadGlobal.vi"("AxisNo"=w279) -> ("AxisWriteValuesOUT"=w278:T5)
                n233 = Bundle By Name(cluster=w278, "AxisStopReq"=TRUE ("AxisWriteValues.AxisMotorON")) -> (w280:T5)
                n234 = call-poly "WriteGloal.vi"("AxisWriteValuesIN"=w280, "AxisNo"=w279) -> ()  [unwired: 1 in]
              }
              frame #1 {
                n235 = Wait (ms)(milliseconds to wait=u32 500) -> ()  [unwired: 1 out]
              }
              frame #2 {
                n236 = call-poly "ReadGlobal.vi"("AxisNo"=w284) -> ("AxisWriteValuesOUT"=w286:T5)
                n237 = Bundle By Name(cluster=w286, "AxisStopReq"=FALSE ("AxisWriteValues.AxisMotorON")) -> (w285:T5)
                n238 = call-poly "WriteGloal.vi"("AxisWriteValuesIN"=w285, "AxisNo"=w284) -> ()  [unwired: 1 in]
              }
            }
          }
        }
      }
      event "StopAppBtn": Value Change {
        n239 = event-data() -> ("OldVal"=w290:bool, "NewVal"=w289:bool)  [unwired: 1 in, 4 out]
        n240 = Not(x=w290) -> (.not. x?=w291:bool)
        n241 = And(x=w291, y=w289) -> (x .and. y?=w288:bool)
        n242 = case shown="True" w288 {
          frame False {
          }
          frame True {
            n243 = property class="App"() -> ("App.Kind"=w292:T10)  [unwired: 2 in, 2 out]
            n244 = case shown="\"Run Time System\"" w292 {
              frame "invalid app kind", Default {
              }
              frame "Run Time System" {
                n245 = Open VI Reference(vi path=path "AxisControl.vi") -> (vi reference=w294:refnum<vi>, error out=w293:errorcluster)  [unwired: 5 in]
                n246 = invoke class="VI" method="FP.Close"(reference=w294, error in=w293) -> ()  [unwired: 1 in, 3 out]
              }
            }
          }
        }
      }
      event "MotorONBtn": Value Change {
        n247 = event-data() -> ("OldVal"=w300:bool, "NewVal"=w298:bool)  [unwired: 1 in, 4 out]
        n248 = Not(x=w300) -> (.not. x?=w299:bool)
        n249 = And(x=w299, y=w298) -> (x .and. y?=w297:bool)
        n250 = case shown="True" w297 {
          tunnel: w296 -> [_ w301]
          frame False {
          }
          frame True {
            # "SIC_STATUS=0 => silnik wyłączony"
            n251 = call-poly "ReadGlobal.vi"("AxisNo"=w301) -> ("AxisReadValuesOUT"=w302:T9)
            n252 = call-poly "ReadGlobal.vi"("AxisNo"=w301) -> ("AxisWriteValuesOUT"=w303:T5)
            n253 = Unbundle By Name(w302) -> ("SICStatus"=w308:i16)
            n254 = Unbundle By Name(w303) -> ("AxisMotorON"=w305:bool)
            n255 = Equal?(x=w308, y=i16 0) -> (x = y?=w306:bool)
            n256 = And(x=w305, y=w306) -> (x .and. y?=w304:bool)
            n257 = case shown="True" w304 {
              tunnel: w301 -> [w309 w315]
              frame False {
                n258 = call-poly "ReadGlobal.vi"("AxisNo"=w309) -> ("AxisWriteValuesOUT"=w311:T5)
                n259 = Bundle By Name(cluster=w311, "AxisMotorON"=TRUE ("AxisWriteValues.AxisMotorON")) -> (w310:T5)
                n260 = call-poly "WriteGloal.vi"("AxisWriteValuesIN"=w310, "AxisNo"=w309) -> ()  [unwired: 1 in]
              }
              frame True {
                n261 = flat-sequence {
                  tunnel: w315 -> [w316]
                  tunnel: [w316] -> w313
                  tunnel: [w320] -> w314
                  tunnel: w313 -> [w320]
                  tunnel: w314 -> [w322]
                  frame #0 {
                    n262 = call-poly "ReadGlobal.vi"("AxisNo"=w316) -> ("AxisWriteValuesOUT"=w318:T5)
                    n263 = Bundle By Name(cluster=w318, "AxisMotorON"=FALSE ("AxisWriteValues.AxisMotorON")) -> (w317:T5)
                    n264 = call-poly "WriteGloal.vi"("AxisWriteValuesIN"=w317, "AxisNo"=w316) -> ()  [unwired: 1 in]
                  }
                  frame #1 {
                    n265 = Wait (ms)(milliseconds to wait=u32 500) -> ()  [unwired: 1 out]
                  }
                  frame #2 {
                    n266 = call-poly "ReadGlobal.vi"("AxisNo"=w322) -> ("AxisWriteValuesOUT"=w324:T5)
                    n267 = Bundle By Name(cluster=w324, "AxisMotorON"=TRUE ("AxisWriteValues.AxisMotorON")) -> (w323:T5)
                    n268 = call-poly "WriteGloal.vi"("AxisWriteValuesIN"=w323, "AxisNo"=w322) -> ()  [unwired: 1 in]
                  }
                }
              }
            }
          }
        }
      }
      event "ReadFileBtn": Value Change {
        n269 = event-data() -> ("OldVal"=w330:bool, "NewVal"=w328:bool)  [unwired: 1 in, 4 out]
        n270 = Not(x=w330) -> (.not. x?=w331:bool)
        n271 = And(x=w331, y=w328) -> (x .and. y?=w327:bool)
        n272 = And(x=w328, y=w327) -> (x .and. y?=w326:bool)
        n273 = case shown="True" w326 {
          tunnel: w329 -> [_ w332]
          frame False {
          }
          frame True {
            n274 = call "File Dialog"("pattern (all files)"="*.ini", "pattern label"="INI files") -> ("selected path"=w334:path, "cancelled"=w335:bool, "error out"=w336:errorcluster)  [unwired: 10 in, 1 out]
            n275 = case shown="False" w335 {
              tunnel: w336 -> [w356 _]
              tunnel: w334 -> [w343 _]
              tunnel: w332 -> [w338 _]
              frame False {
                n276 = call <vilib>:"Application Directory.vi"() -> ("Application Directory"=w348:path)
                n277 = call-poly "ReadGlobal.vi"("AxisNo"=w338) -> ("AxisConfigurationOUT"=w340:T2)
                n278 = Build Path(base path=w348, name or relative path="SMCD14AxisControl.ini") -> (appended path=w349:path)
                n279 = call-poly "ReadGlobal.vi"("AxisNo"=w338) -> ("AxisWriteValuesOUT"=w339:T5)
                n280 = call <vilib>:"Open Config Data.vi"("create file if necessary (T)"=FALSE, "configuration file path"=w349) -> ("error out"=w351:errorcluster, "refnum"=w350:T1)  [unwired: 7 in, 1 out]
                n281 = Strip Path(path=w343) -> (name=w352:string)  [unwired: 1 out]
                n282 = call-poly <vilib>:"Write Key.vi"("section"="default", "error in (no error)"=w351, "value"=w352, "key"="ConfigFile", "refnum"=w350) -> ("error out"=w354:errorcluster, "refnum out"=w353:T1)  [unwired: 4 in, 1 out]
                n283 = call "AxisGetConfFromFile.vi"("conf file path"=w343, "error in (no error)"=w356, "AxisWriteValuesIn"=w339, "AxisConfigurationIn"=w340) -> ("error out"=w355:errorcluster, "AditionalConfigOut"=w342:T3, "AxisWriteValuesOut"=w358:T5, "AxisConfigurationOut"=w357:T2, "Comunication"=w341:T4)  [unwired: 3 in]
                n284 = call <vilib>:"Close Config Data.vi"("error in (no error)"=w354, "refnum"=w353) -> ()  [unwired: 8 in, 2 out]
                n285 = case shown="No Error" w355 {
                  tunnel: w358 -> [w360 _]
                  tunnel: w357 -> [w362 _]
                  tunnel: w342 -> [w371 _]
                  tunnel: w341 -> [w370 _]
                  tunnel: w338 -> [w361 _]
                  frame No Error {
                    n286 = Unbundle By Name(w362) -> ("AxisName"=w377:string, "AxisUnit"=w376:u16, "AxisHomeType"=w375:u16, "AxisBacklash"=w374:dbl, "AxisGain"=w373:dbl, "AxisOffset"=w372:dbl)
                    n287 = Unbundle By Name(w360) -> ("AxisHomingVel"=w379:dbl, "AxisAccDecc"=w378:dbl)
                    n288 = Unbundle By Name(w371) -> ("Joy_slow_speed"=w367:sgl, "Joy_slow_fast"=w368:sgl, "MaxVel"=w369:sgl, "Joystick_control"=w359:bool)  [unwired: 2 out]
                    n289 = Unbundle By Name(w370) -> ("DeviceIDCtrl"=w366:u16, "ProtocolCtrl"=w363:enum16{"Modbus RTU", "Modbus TCP", ""}, "COMportCtrl"=w364:refnum<visa-resource-name>, "IPCtrl"=w365:string)
                    n290 = property on="AxisName" class="Str"("Value"=w377) -> ()  [unwired: 2 in, 2 out]
                    n291 = property on="UnitsControl" class="Ring (strict)"("Value"=w376) -> ()  [unwired: 2 in, 2 out]
                    n292 = property on="HomingTypeControl" class="Ring (strict)"("Value"=w375) -> ()  [unwired: 2 in, 2 out]
                    n293 = property on="BacklashControl" class="DigNum (strict)"("Value"=w374) -> ()  [unwired: 2 in, 2 out]
                    n294 = property on="GainControl" class="DigNum (strict)"("Value"=w373) -> ()  [unwired: 2 in, 2 out]
                    n295 = property on="OffsetControl" class="DigNum (strict)"("Value"=w372) -> ()  [unwired: 2 in, 2 out]
                    n296 = property on="HomingVelControl" class="DigNum (strict)"("Value"=w379) -> ()  [unwired: 2 in, 2 out]
                    n297 = property on="AccDeccControl" class="DigNum (strict)"("Value"=w378) -> ()  [unwired: 2 in, 2 out]
                    n298 = local write "JoyMinSpeed"(w367) -> ()
                    n299 = local write "JoyMaxSpeed"(w368) -> ()
                    n300 = local write "Max Velocity"(w369) -> ()
                    n301 = local write "Joystick control"(w359) -> ()
                    n302 = local write "ProtocolCtrl"(w366) -> ()
                    n303 = local write "DeviceIDCtrl"(w363) -> ()
                    n304 = local write "COMportCtrl"(w364) -> ()
                    n305 = local write "IPCtrl"(w365) -> ()
                    n306 = call-poly "WriteGloal.vi"("AxisConfigurationIN"=w362, "AxisNo"=w361) -> ()  [unwired: 1 in]
                    n307 = call-poly "WriteGloal.vi"("AxisWriteValuesIN"=w360, "AxisNo"=w361) -> ()  [unwired: 1 in]
                  }
                  frame Error {
                  }
                }
              }
              frame True {
              }
            }
          }
        }
      }
      event "WriteFileBtn": Value Change {
        n308 = event-data() -> ("OldVal"=w384:bool, "NewVal"=w381:bool)  [unwired: 1 in, 4 out]
        n309 = Not(x=w384) -> (.not. x?=w385:bool)
        n310 = And(x=w385, y=w381) -> (x .and. y?=w382:bool)
        n311 = And(x=w382, y=w381) -> (x .and. y?=w380:bool)
        n312 = case shown="True" w380 {
          tunnel: w383 -> [_ w386]
          frame False {
          }
          frame True {
            n313 = call "File Dialog2"("pattern (all files)"="*.ini", "pattern label"="INI files") -> ("selected path"=w387:path, "cancelled"=w400:bool, "error out"=w399:errorcluster)  [unwired: 10 in, 1 out]
            n314 = call <vilib>:"Application Directory.vi"() -> ("Application Directory"=w392:path)
            n315 = Build Path(base path=w392, name or relative path="SMCD14AxisControl.ini") -> (appended path=w393:path)
            n316 = call <vilib>:"Open Config Data.vi"("create file if necessary (T)"=FALSE, "configuration file path"=w393) -> ("error out"=w395:errorcluster, "refnum"=w394:T1)  [unwired: 7 in, 1 out]
            n317 = Strip Path(path=w387) -> (name=w396:string)  [unwired: 1 out]
            n318 = call-poly <vilib>:"Write Key.vi"("section"="default", "error in (no error)"=w395, "value"=w396, "key"="ConfigFile", "refnum"=w394) -> ("error out"=w398:errorcluster, "refnum out"=w397:T1)  [unwired: 4 in, 1 out]
            n319 = call <vilib>:"Close Config Data.vi"("error in (no error)"=w398, "refnum"=w397) -> ()  [unwired: 8 in, 2 out]
            n320 = case shown="False" w400 {
              tunnel: w387 -> [w428 _]
              tunnel: w399 -> [w427 _]
              tunnel: w386 -> [w403 _]
              frame False {
                n321 = call-poly "ReadGlobal.vi"("AxisNo"=w403) -> ("AxisWriteValuesOUT"=w404:T5)
                n322 = local read "Max Velocity"() -> (w407:dbl)
                n323 = local read "JoyMaxSpeed"() -> (w414:dbl)
                n324 = local read "JoyMinSpeed"() -> (w406:dbl)
                n325 = call-poly "ReadGlobal.vi"("AxisNo"=w403) -> ("AxisConfigurationOUT"=w405:T2)
                n326 = local read "HomingTypeControl"() -> (w425:u16)
                n327 = local read "HomingVelControl"() -> (w421:dbl)
                n328 = local read "BacklashControl"() -> (w424:dbl)
                n329 = local read "AccDeccControl"() -> (w420:dbl)
                n330 = local read "OffsetControl"() -> (w422:dbl)
                n331 = local read "UnitsControl"() -> (w413:u16)
                n332 = local read "GainControl"() -> (w423:dbl)
                n333 = local read "AxisName"() -> (w412:string)
                n334 = Bundle By Name(cluster=T7 {"Joy_slow_speed"=0.0, "Joy_slow_fast"=0.0, "Name"="", "UnitsControl"=0, "MaxVel"=0.0} ("Cluster"), "Joy_slow_speed"=w406, "Joy_slow_fast"=w414, "Name"=w412, "UnitsControl"=w413, "MaxVel"=w407) -> (w416:T7)
                n335 = Bundle By Name(cluster=w405, "AxisHomeType"=w425, "AxisBacklash"=w424, "AxisGain"=w423, "AxisOffset"=w422, "AxisUnit"=w413, "AxisName"=w412) -> (w426:T2)
                n336 = local read "COMportCtrl"() -> (w411:refnum<visa-resource-name>)
                n337 = local read "DeviceIDCtrl"() -> (w409:u16)
                n338 = local read "ProtocolCtrl"() -> (w410:u16)
                n339 = Bundle By Name(cluster=w404, "AxisHomingVel"=w421, "AxisAccDecc"=w420) -> (w419:T5)
                n340 = local read "IPCtrl"() -> (w408:string)
                n341 = Bundle By Name(cluster=T4 {"DeviceIDCtrl"=1, "ProtocolCtrl"=enum."Modbus RTU", "COMportCtrl"="", "IPCtrl"=""} ("Comunication 2"), "DeviceIDCtrl"=w409, "ProtocolCtrl"=w410, "COMportCtrl"=w411, "IPCtrl"=w408) -> (w415:T4)
                n342 = call "AxisSaveConfToFile.vi"("Comunication"=w415, "conf file path"=w428, "error in (no error)"=w427, "AditionalConfigOut"=w416, "AxisWriteValuesIn"=w419, "AxisConfigurationIn"=w426) -> ()  [unwired: 5 in, 1 out]
              }
              frame True {
              }
            }
          }
        }
      }
      event "MotorOFFBtn": Value Change {
        n343 = event-data() -> ("OldVal"=w433:bool, "NewVal"=w431:bool)  [unwired: 1 in, 4 out]
        n344 = Not(x=w433) -> (.not. x?=w432:bool)
        n345 = And(x=w432, y=w431) -> (x .and. y?=w430:bool)
        n346 = case shown="True" w430 {
          tunnel: w429 -> [_ w434]
          frame False {
          }
          frame True {
            n347 = call-poly "ReadGlobal.vi"("AxisNo"=w434) -> ("AxisWriteValuesOUT"=w436:T5)
            n348 = Bundle By Name(cluster=w436, "AxisMotorON"=FALSE ("AxisWriteValues.AxisMotorON")) -> (w435:T5)
            n349 = call-poly "WriteGloal.vi"("AxisWriteValuesIN"=w435, "AxisNo"=w434) -> ()  [unwired: 1 in]
          }
        }
      }
      event "TargetControl": Value Change {
        n350 = event-data() -> ("NewVal"=w441:dbl)  [unwired: 1 in, 5 out]
        n351 = call-poly "ReadGlobal.vi"("AxisNo"=w439) -> ("AxisWriteValuesOUT"=w440:T5)
        n352 = Bundle By Name(cluster=w440, "AxisTarget"=w441) -> (w438:T5)
        n353 = call-poly "WriteGloal.vi"("AxisWriteValuesIN"=w438, "AxisNo"=w439) -> ()  [unwired: 1 in]
      }
      event "AccDeccControl": Value Change {
        n354 = event-data() -> ("NewVal"=w445:dbl)  [unwired: 1 in, 5 out]
        n355 = call-poly "ReadGlobal.vi"("AxisNo"=w443) -> ("AxisWriteValuesOUT"=w444:T5)
        n356 = Bundle By Name(cluster=w444, "AxisAccDecc"=w445) -> (w442:T5)
        n357 = call-poly "WriteGloal.vi"("AxisWriteValuesIN"=w442, "AxisNo"=w443) -> ()  [unwired: 1 in]
      }
      event "AxisName": Value Change {
        n358 = event-data() -> ("NewVal"=w449:string)  [unwired: 1 in, 5 out]
        n359 = call-poly "ReadGlobal.vi"("AxisNo"=w447) -> ("AxisConfigurationOUT"=w448:T2)
        n360 = Bundle By Name(cluster=w448, "AxisName"=w449) -> (w446:T2)
        n361 = call-poly "WriteGloal.vi"("AxisConfigurationIN"=w446, "AxisNo"=w447) -> ()  [unwired: 1 in]
      }
      event "UnitsControl": Value Change {
        n362 = event-data() -> ("NewVal"=w453:u16)  [unwired: 1 in, 5 out]
        n363 = call-poly "ReadGlobal.vi"("AxisNo"=w451) -> ("AxisConfigurationOUT"=w452:T2)
        n364 = Bundle By Name(cluster=w452, "AxisUnit"=w453) -> (w450:T2)
        n365 = call-poly "WriteGloal.vi"("AxisConfigurationIN"=w450, "AxisNo"=w451) -> ()  [unwired: 1 in]
      }
      event "HomingTypeControl": Value Change {
        n366 = event-data() -> ("NewVal"=w457:u16)  [unwired: 1 in, 5 out]
        n367 = call-poly "ReadGlobal.vi"("AxisNo"=w455) -> ("AxisConfigurationOUT"=w456:T2)
        n368 = Bundle By Name(cluster=w456, "AxisHomeType"=w457) -> (w454:T2)
        n369 = call-poly "WriteGloal.vi"("AxisConfigurationIN"=w454, "AxisNo"=w455) -> ()  [unwired: 1 in]
      }
      event "HomingVelControl": Value Change {
        n370 = event-data() -> ("NewVal"=w461:dbl)  [unwired: 1 in, 5 out]
        n371 = call-poly "ReadGlobal.vi"("AxisNo"=w459) -> ("AxisWriteValuesOUT"=w460:T5)
        n372 = Bundle By Name(cluster=w460, "AxisHomingVel"=w461) -> (w458:T5)
        n373 = call-poly "WriteGloal.vi"("AxisWriteValuesIN"=w458, "AxisNo"=w459) -> ()  [unwired: 1 in]
      }
      event "VelocityControl": Value Change {
        n374 = event-data() -> ("NewVal"=w465:dbl)  [unwired: 1 in, 5 out]
        n375 = call-poly "ReadGlobal.vi"("AxisNo"=w463) -> ("AxisWriteValuesOUT"=w464:T5)
        n376 = Bundle By Name(cluster=w464, "AxisTargetVel"=w465) -> (w462:T5)
        n377 = call-poly "WriteGloal.vi"("AxisWriteValuesIN"=w462, "AxisNo"=w463) -> ()  [unwired: 1 in]
      }
      event "MoveModeControl": Value Change {
        n378 = event-data() -> ("NewVal"=w469:u16)  [unwired: 1 in, 5 out]
        n379 = call-poly "ReadGlobal.vi"("AxisNo"=w467) -> ("AxisWriteValuesOUT"=w468:T5)
        n380 = Bundle By Name(cluster=w468, "MoveModeControl"=w469) -> (w466:T5)
        n381 = call-poly "WriteGloal.vi"("AxisWriteValuesIN"=w466, "AxisNo"=w467) -> ()  [unwired: 1 in]
      }
    }
    n382 = local read "StopAppBtn"() -> (w84:bool)
  }
  n383 = while "IndicatorsRefresh" {
    stop <- w496 stop-if-true
    w487 = i16 0 ("x")
    n384 = local read "SubPanelNo"() -> (w471:u16)
    n385 = call-poly "ReadGlobal.vi"("AxisNo"=w471) -> ("AxisWriteValuesOUT"=w473:T5)
    n386 = call-poly "ReadGlobal.vi"("AxisNo"=w471) -> ("ConnectionDataOUT"=w474:T8)
    n387 = call-poly "ReadGlobal.vi"("AxisNo"=w471) -> ("AxisReadValuesOUT"=w472:T9)
    n388 = call-poly "ReadGlobal.vi"("AxisNo"=w471) -> ("ConnectionDataOUT"=w475:T8)
    n389 = case shown="\"Axis\"" "MainTabs" {
      tunnel: w471 -> [w508 w546 _]
      frame "Axis" {
        n390 = local read "IsSubPanel"() -> (w510:bool)
        n391 = case shown="True" w510 {
          tunnel: [w536 w541] -> w517
          tunnel: [w537 w540] -> w514
          tunnel: w508 -> [_ w538]
          frame True {
            n392 = local read "AxisName"() -> (w537:string)
            n393 = local read "UnitsControl"() -> (w536:u16)
          }
          frame False {
            n394 = call-poly "ReadGlobal.vi"("AxisNo"=w538) -> ("AxisConfigurationOUT"=w539:T2)
            n395 = Unbundle By Name(w539) -> ("AxisUnit"=w541:u16, "AxisName"=w540:string)
          }
        }
        n396 = call-poly "ReadGlobal.vi"("AxisNo"=w508) -> ("AxisReadValuesOUT"=w509:T9)
        n397 = Unbundle By Name(w509) -> ("AxisPosition"=→"AxisPosIndicator":dbl, "AxisInPos"=→"InPosIndicator":bool, "AxisRun"=→"IsRunningIndicator":bool, "AxisHomed"=→"IsHomedIndicator":bool, "AxisFLS"=→"FLSIndicator":bool, "AxisBLS"=→"BLSIndicator":bool, "AxisEnabled"=→"EnabledIndicator":bool, "AxisError"=→"ErrorIndicator":bool, "AxisDog"=→"RefIndicator":bool, "AxisErrorCode"=w527:i16, "AxisVelocity"=→"AxisVelIndicator":dbl, "AxisMotorON"=→"MotorIndicator":bool)  [unwired: 1 out]
        n398 = case shown="0, Default" w517 {
          tunnel: ["[mm]" ("string") "[°]" ("string")] -> w519
          tunnel: ["[mm/s]" ("string") "[°/s]" ("string")] -> w518
          frame 0, Default {
          }
          frame 1 {
          }
        }
        n399 = Concatenate Strings(w514, " Axis Control" ("string")) -> (w513:string)
        n400 = Concatenate Strings(w514, " Axis Status" ("string")) -> (w512:string)
        n401 = call "ErrorDescription.vi"("AxisReadValues.AxisErrorCode"=w527) -> ("ErrorDescription"=→"ErrorCodeIndicator":string)
        n402 = Concatenate Strings("Position " ("string"), w519) -> (w522:string)
        n403 = Concatenate Strings("Velocity " ("string"), w518) -> (w521:string)
        n404 = property on="AxisControlFrame" class="SubPnl"("Caption.Text"=w513) -> ()  [unwired: 2 in, 2 out]
        n405 = property on="AxisStatusFrame" class="SubPnl"("Caption.Text"=w512) -> ()  [unwired: 2 in, 2 out]
        n406 = property on="AxisPosIndicator" class="DigNum (strict)"("Caption.Text"=w522) -> ()  [unwired: 2 in, 2 out]
        n407 = property on="AxisVelIndicator" class="DigNum (strict)"("Caption.Text"=w521) -> ()  [unwired: 2 in, 2 out]
      }
      frame "Connection", Default {
        n408 = call-poly "ReadGlobal.vi"("AxisNo"=w546) -> ("ConnectionDataOUT"=w547:T8)
        n409 = Unbundle By Name(w547) -> ("ConnectionStatusIndicator"=w549:bool)
        n410 = case shown="False" w549 {
          tunnel: ["Connect" ("ConnectionStatusIndicator") "Disconnect" ("ConnectionStatusIndicator")] -> w548
          frame False {
          }
          frame True {
          }
        }
        n411 = property on="ConnectBtn" class="Bool (strict)"("BoolText.Text"=w548) -> ()  [unwired: 2 in, 2 out]
      }
      frame "Config." {
      }
    }
    n412 = Wait Until Next ms Multiple(millisecond multiple=u32 50) -> ()  [unwired: 1 out]
    n413 = Unbundle By Name(w473) -> ("MoveModeControl"=w478:u16, "AxisTargetVel"=w488:dbl)
    n414 = Unbundle By Name(w472) -> ("SICStatus"=w490:i16, "AxisErrorCode"=w489:i16, "AxisEnabled"=w483:bool)
    n415 = Unbundle By Name(w474) -> ("ConnectionStatusIndicator"=w486:bool)
    n416 = Unbundle By Name(w475) -> ("ConnectionStatusIndicator"=w494:bool)
    n417 = Not Equal?(x=w487, y=w490) -> (x != y?=w485:bool)
    n418 = Equal?(x=w487, y=w489) -> (x = y?=w484:bool)
    n419 = Not Equal?(x=w487, y=w478) -> (x != y?=w482:bool)
    n420 = Not Equal?(x=w487, y=w488) -> (x != y?=w480:bool)
    n421 = Equal?(x=w478, y=u16 4) -> (x = y?=w476:bool)
    n422 = case shown="True" w494 {
      tunnel: ["Not connected" ("ConnectionStatusIndicator") "Connected" ("ConnectionStatusIndicator")] -> w493
      tunnel: [TRUE ("Text.Font:Bold") TRUE ("Text.Font:Bold")] -> w492
      tunnel: ["Connect" ("Boolean Text.Text") "Disconnect" ("Boolean Text.Text")] -> w491
      tunnel: [T11 {"Text Color"=0, "Background Color"=16711680} ("Text.Text Colors") T11 {"Text Color"=0, "Background Color"=6618880} ("Text.Text Colors")] -> w470
      frame False {
      }
      frame True {
      }
    }
    "ConnectionStatusIndicator" <- w493
    n423 = Or(x=w480, y=w476) -> (x .or. y?=w479:bool)
    n424 = Compound Arithmetic op=AND(w486, w485, w484, w483, w482, w479) -> (w481:bool)
    n425 = case shown="False" w481 {
      frame False {
        n426 = property on="RunBtn" class="Bool (strict)"("DisabledEnum"=T6."Disabled and Grayed Out" ("Disabled")) -> ()  [unwired: 2 in, 2 out]
      }
      frame True {
        n427 = property on="RunBtn" class="Bool (strict)"("DisabledEnum"=T6."Enabled" ("Disabled")) -> ()  [unwired: 2 in, 2 out]
      }
    }
    n428 = local read "StopAppBtn"() -> (w496:bool)
    n429 = property on="ConnectBtn2" class="Bool (strict)"("BoolText.Text"=w491) -> ()  [unwired: 2 in, 2 out]
    n430 = property on="ConnectionStatusIndicator" class="Str"("Text.FontBold"=w492) -> ()  [unwired: 2 in, 2 out]
    n431 = property on="ConnectionStatusIndicator" class="Str"("Text.TextColors"=w470) -> ()  [unwired: 2 in, 2 out]
  }
  n432 = while "ModbusOperations" {
    i -> [w552]
    stop <- w556 stop-if-true
    n433 = local read "SubPanelNo"() -> (w553:u16)
    n434 = local read "StopAppBtn"() -> (w556:bool)
    n435 = call-poly "ReadGlobal.vi"("AxisNo"=w553) -> ("ConnectionDataOUT"=w554:T8)
    n436 = Wait Until Next ms Multiple(millisecond multiple=u32 250) -> ()  [unwired: 1 out]
    n437 = Unbundle By Name(w554) -> ("ConnectionStatusIndicator"=w555:bool)
    n438 = case shown="True" w555 {
      tunnel: w553 -> [_ w559]
      tunnel: w552 -> [_ w558]
      frame False {
      }
      frame True {
        n439 = flat-sequence {
          tunnel: [w573] -> w563
          tunnel: w559 -> [w569]
          tunnel: w558 -> [w568]
          tunnel: [w586] -> w564
          tunnel: w563 -> [w586]
          tunnel: w564 -> [w591]
          tunnel: [w590] -> w562
          tunnel: w559 -> [w588]
          tunnel: w562 -> [w602]
          tunnel: [w601] -> w561
          tunnel: w559 -> [w599]
          tunnel: w561 -> [w639]
          tunnel: [w638] -> w560
          tunnel: w559 -> [w636]
          frame #0 {
            # "Stały odczy nazwy i jednostki:"
            # "Odczytywanie rejestrów"
            n440 = call-poly "ReadGlobal.vi"("AxisNo"=w569) -> ("ConnectionDataOUT"=w571:T8)
            n441 = Unbundle By Name(w571) -> ("serial master instance"=w574:refnum<class "Modbus Master.lvclass">)
            n442 = Quotient & Remainder(x=w568, y=16) -> (x-y*floor(x/y)=w566:i32)  [unwired: 1 out]
            n443 = Equal To 0?(x=w566) -> (x = 0?=w565:bool)
            n444 = call "AxisFetchRegs.vi"("read aditional data"=w565, "Modbus master"=w574) -> ("error out"=w573:errorcluster, "JoyControl"=w572:T3, "AxisReadValues"=w570:T9)  [unwired: 7 in]
            n445 = case shown="True" w565 {
              tunnel: w572 -> [_ w583]
              tunnel: w569 -> [_ w576]
              frame False {
              }
              frame True {
                n446 = Unbundle By Name(w583) -> ("Name"=w578:string, "UnitsControl"=w579:u16, "MaxVel"=w580:sgl)  [unwired: 2 out]
                n447 = Greater Or Equal?(x=w580, y=0.0) -> (x >= y?=w581:bool)
                n448 = case shown="True" w581 {
                  tunnel: w580 -> [_ w584]
                  frame False {
                  }
                  frame True {
                    n449 = Negate(x=w584) -> (-x=w585:sgl)
                    n450 = property on="VelocityControl" class="DigNum (strict)"("Maximum"=w584, "Minimum"=w585) -> ()  [unwired: 2 in, 2 out]
                  }
                }
                n451 = call-poly "ReadGlobal.vi"("AxisNo"=w576) -> ("AxisConfigurationOUT"=w577:T2)
                n452 = Bundle By Name(cluster=w577, "AxisUnit"=w579, "AxisName"=w578) -> (w575:T2)
                n453 = call-poly "WriteGloal.vi"("AxisConfigurationIN"=w575, "AxisNo"=w576) -> ()  [unwired: 1 in]
              }
            }
            n454 = call-poly "WriteGloal.vi"("AxisReadValuesIN"=w570, "AxisNo"=w569) -> ()  [unwired: 1 in]
          }
          frame #1 {
            # "było 50"
            # "Chwila przerwy"
            n455 = Wait (ms)(milliseconds to wait=u32 2) -> ()  [unwired: 1 out]
          }
          frame #2 {
            # "Zapisywanie rejestrów"
            n456 = local read "ReadOnlyMode"() -> (w589:bool)
            n457 = case shown="False" w589 {
              tunnel: w591 -> [w597 w598]
              tunnel: [w596 w598] -> w590
              tunnel: w588 -> [w592 _]
              frame False {
                n458 = call-poly "ReadGlobal.vi"("AxisNo"=w592) -> ("ConnectionDataOUT"=w594:T8)
                n459 = Unbundle By Name(w594) -> ("serial master instance"=w595:refnum<class "Modbus Master.lvclass">)
                n460 = call-poly "ReadGlobal.vi"("AxisNo"=w592) -> ("AxisWriteValuesOUT"=w593:T5)
                n461 = call "AxisWriteRegs.vi"("error in"=w597, "AxisWriteValues"=w593, "Modbus master"=w595) -> ("error out"=w596:errorcluster)  [unwired: 8 in]
              }
              frame True {
              }
            }
          }
          frame #3 {
            # "Ewentualnie odczyt konfiguracji, jeśli trzeba"
            n462 = call-poly "ReadGlobal.vi"("AxisNo"=w599) -> ("AxisConfigurationOUT"=w600:T2)
            n463 = Unbundle By Name(w600) -> ("ReqConfRead"=w603:bool)
            n464 = case shown="True" w603 {
              tunnel: w602 -> [w604 w620]
              tunnel: [w604 w619] -> w601
              tunnel: w599 -> [_ w607]
              frame False {
              }
              frame True {
                n465 = call-poly "ReadGlobal.vi"("AxisNo"=w607) -> ("ConnectionDataOUT"=w608:T8)
                n466 = flat-sequence {
                  tunnel: w625 -> [w628]
                  tunnel: w607 -> [w627]
                  tunnel: [w627] -> w606
                  tunnel: w610 -> [w632]
                  tunnel: w609 -> [w633]
                  tunnel: w606 -> [w629]
                  frame #0 {
                    n467 = call-poly "WriteGloal.vi"("AxisConfigurationIN"=w628, "AxisNo"=w627) -> ()  [unwired: 1 in]
                  }
                  frame #1 {
                    n468 = local write "UnitsControl"(w632) -> ()
                    n469 = call-poly "ReadGlobal.vi"("AxisNo"=w629) -> ("AxisConfigurationOUT"=w630:T2)
                    n470 = Bundle By Name(cluster=w630, "AxisUnit"=w632, "AxisName"=w633) -> (w631:T2)
                    n471 = call-poly "WriteGloal.vi"("AxisConfigurationIN"=w631, "AxisNo"=w629) -> ()  [unwired: 1 in]
                  }
                }
                n472 = Unbundle By Name(w608) -> ("serial master instance"=w626:refnum<class "Modbus Master.lvclass">)
                n473 = call "AxisFetchConf.vi"("error in"=w620, "Modbus master"=w626) -> ("error out"=w619:errorcluster, "JoyControl"=w611:T3, "AxisConfiguration"=w625:T2)  [unwired: 7 in]
                n474 = Unbundle By Name(w625) -> ("AxisHomeType"=w624:u16, "AxisBacklash"=w623:dbl, "AxisGain"=w622:dbl, "AxisOffset"=w621:dbl, "AxisAccDecc"=w618:dbl, "AxisHomeVel"=w617:dbl)
                n475 = Unbundle By Name(w611) -> ("Joy_slow_speed"=w614:sgl, "Joy_slow_fast"=w613:sgl, "Name"=w609:string, "UnitsControl"=w610:u16, "MaxVel"=w616:sgl, "Joystick_control"=w605:bool)
                n476 = local write "HomingVelControl"(w617) -> ()
                n477 = local write "HomingTypeControl"(w624) -> ()
                n478 = Greater Or Equal?(x=w616, y=0.0) -> (x >= y?=w615:bool)
                n479 = case shown="True" w615 {
                  tunnel: w616 -> [_ w634]
                  frame False {
                  }
                  frame True {
                    n480 = Negate(x=w634) -> (-x=w635:sgl)
                    n481 = property on="VelocityControl" class="DigNum (strict)"("Maximum"=w634, "Minimum"=w635) -> ()  [unwired: 2 in, 2 out]
                    n482 = local write "Max Velocity"(w634) -> ()
                  }
                }
                n483 = local write "BacklashControl"(w623) -> ()
                n484 = local write "AccDeccControl"(w618) -> ()
                n485 = local write "OffsetControl"(w621) -> ()
                n486 = local write "GainControl"(w622) -> ()
                n487 = local write "JoyMinSpeed"(w614) -> ()
                n488 = local write "JoyMaxSpeed"(w613) -> ()
                n489 = local write "Joystick control"(w605) -> ()
                n490 = property on="AxisName" class="Str"("Value"=w609) -> ()  [unwired: 2 in, 2 out]
              }
            }
          }
          frame #4 {
            # "Ewentualnie zapis konfiguracji, jeśli trzeba"
            n491 = local read "ReadOnlyMode"() -> (w637:bool)
            n492 = case shown="False" w637 {
              tunnel: w639 -> [w643 w668]
              tunnel: [w642 w668] -> w638
              tunnel: w636 -> [w640 _]
              frame False {
                n493 = call-poly "ReadGlobal.vi"("AxisNo"=w640) -> ("AxisConfigurationOUT"=w641:T2)
                n494 = Unbundle By Name(w641) -> ("ReqConfWrite"=w644:bool)
                n495 = case shown="True" w644 {
                  tunnel: w641 -> [_ w666]
                  tunnel: w643 -> [w645 w660]
                  tunnel: [w645 w659] -> w642
                  tunnel: w640 -> [_ w648]
                  frame False {
                  }
                  frame True {
                    n496 = local read "HomingVelControl"() -> (w657:dbl)
                    n497 = local read "AccDeccControl"() -> (w658:dbl)
                    n498 = local read "OffsetControl"() -> (w662:dbl)
                    n499 = local read "Joystick control"() -> (w646:bool)
                    n500 = local read "HomingTypeControl"() -> (w665:u16)
                    n501 = local read "JoyMaxSpeed"() -> (w655:dbl)
                    n502 = local read "JoyMinSpeed"() -> (w656:dbl)
                    n503 = local read "Max Velocity"() -> (w652:dbl)
                    n504 = local read "UnitsControl"() -> (w653:u16)
                    n505 = local read "GainControl"() -> (w663:dbl)
                    n506 = local read "BacklashControl"() -> (w664:dbl)
                    n507 = local read "AxisName"() -> (w654:string)
                    n508 = call-poly "ReadGlobal.vi"("AxisNo"=w648) -> ("ConnectionDataOUT"=w650:T8)
                    n509 = Bundle By Name(cluster=w666, "AxisHomeType"=w665, "AxisBacklash"=w664, "AxisGain"=w663, "AxisOffset"=w662, "AxisAccDecc"=w658, "AxisHomeVel"=w657) -> (w661:T2)
                    n510 = Unbundle By Name(w650) -> ("serial master instance"=w667:refnum<class "Modbus Master.lvclass">)
                    n511 = Bundle By Name(cluster=T3 {"Joy_slow_speed"=0.0, "Joy_slow_fast"=0.0, "Name"="", "UnitsControl"=0, "MaxVel"=0.0, "Joystick_control"=FALSE} ("JoyControl"), "Joy_slow_speed"=w656, "Joy_slow_fast"=w655, "Name"=w654, "UnitsControl"=w653, "MaxVel"=w652, "Joystick_control"=w646) -> (w651:T3)
                    n512 = call "AxisWriteConf.vi"("AditionalConfig"=w651, "error in"=w660, "AxisConfigurationIn"=w661, "Modbus master"=w667) -> ("error out"=w659:errorcluster, "AxisConfigurationOut"=w649:T2)  [unwired: 6 in]
                    n513 = call-poly "WriteGloal.vi"("AxisConfigurationIN"=w649, "AxisNo"=w648) -> ()  [unwired: 1 in]
                  }
                }
              }
              frame True {
              }
            }
          }
        }
        n514 = case shown="Error" w560 {
          selector: w560 -> [_ w669]
          tunnel: w559 -> [_ w670]
          frame No Error {
          }
          frame Error {
            n515 = call-poly "ReadGlobal.vi"("AxisNo"=w670) -> ("ConnectionDataOUT"=w671:T8)
            n516 = Unbundle By Name(w671) -> ("ConnectionStatusIndicator"=w672:bool)
            n517 = case shown="True" w672 {
              tunnel: w670 -> [_ w674]
              tunnel: w669 -> [_ _]
              frame False {
              }
              frame True {
                n518 = call-poly "ReadGlobal.vi"("AxisNo"=w674) -> ("ConnectionDataOUT"=w675:T8)
                n519 = Bundle By Name(cluster=w675, "ConnectionStatusIndicator"=FALSE) -> (w673:T8)
                n520 = One Button Dialog(message="Communication error!\nError while reading/writing to device.") -> ()  [unwired: 1 in, 1 out]
                n521 = call-poly "WriteGloal.vi"("ConnectionDataIN"=w673, "AxisNo"=w674) -> ()  [unwired: 1 in]
              }
            }
          }
        }
      }
    }
  }
  n522 = while "Heartbeat monitor" {
    shift-right: [w684] -> _
    shift-left: _ -> [w683]
    shift-right: [w685] -> _
    shift-left: _ -> [w686]
    stop <- w688 stop-if-true
    n523 = local read "SubPanelNo"() -> (w678:u16)
    n524 = call-poly "ReadGlobal.vi"("AxisNo"=w678) -> ("ConnectionDataOUT"=w679:T8)
    n525 = Unbundle By Name(w679) -> ("ConnectionStatusIndicator"=w682:bool)
    n526 = local read "CheckProg"() -> (w680:bool)
    n527 = And(x=w680, y=w682) -> (x .and. y?=w681:bool)
    n528 = case shown="False" w681 {
      tunnel: w686 -> [w689 w697]
      tunnel: [w689 w696] -> w685
      tunnel: [w690 w694] -> w684
      tunnel: w683 -> [w690 w693]
      tunnel: w678 -> [_ w691]
      frame False {
      }
      frame True {
        n529 = call-poly "ReadGlobal.vi"("AxisNo"=w691) -> ("AxisReadValuesOUT"=w692:T9)
        n530 = Unbundle By Name(w692) -> ("AxisHeartbeat"=w696:i16)
        n531 = Equal?(x=w696, y=w697) -> (x = y?=w695:bool)
        n532 = case shown="True" w695 {
          tunnel: [0 w700] -> w694
          tunnel: w693 -> [_ w701]
          tunnel: w691 -> [_ w699]
          frame False {
          }
          frame True {
            n533 = Greater?(x=w701, y=25) -> (0:w702:bool)
            n534 = case shown="True" w702 {
              tunnel: w701 -> [w706 _]
              tunnel: [w704 0] -> w700
              tunnel: w699 -> [_ w707]
              frame False {
                n535 = Add(x=w706, y=1) -> (x+y=w704:i32)
              }
              frame True {
                n536 = call-poly "ReadGlobal.vi"("AxisNo"=w707) -> ("ConnectionDataOUT"=w709:T8)
                n537 = Bundle By Name(cluster=w709, "ConnectionStatusIndicator"=FALSE) -> (w708:T8)
                n538 = call-poly "WriteGloal.vi"("ConnectionDataIN"=w708, "AxisNo"=w707) -> ()  [unwired: 1 in]
                n539 = One Button Dialog(message="SMCD14 device not found. Possible reasons:\n- connected other modbus device\n- SMCD14 user program stopped or program error") -> ()  [unwired: 1 in, 1 out]
              }
            }
          }
        }
      }
    }
    n540 = local read "StopAppBtn"() -> (w688:bool)
    n541 = Wait Until Next ms Multiple(millisecond multiple=u32 1000) -> ()  [unwired: 1 out]
  }
